vi "Generate.vi"(8 "error in (no error)":errorcluster, 10 "PCL Rate (secs)":dbl, 11 "Frame Configurations":T1[](array[typedef]) {"CD Results Refs"."Data Reference" format="%.0x"; "Input Channels Refs"."Data Reference" format="%.0x"; "Frame Configuration"."CRC"."Data Type" items=["Signed", "Unsigned", "IEEE Float"]; "Frame Configuration"."Rolling Counter"."Data Type" items=["Signed", "Unsigned", "IEEE Float"]; "Frame Configuration"."Input Channels"."Data Type" items=["Signed", "Unsigned", "IEEE Float"]}) -> (0 "error out":errorcluster, 3 "Frame Configurations":T1[](array[typedef]) {"CD Results Refs"."Data Reference" format="%.0x"; "Input Channels Refs"."Data Reference" format="%.0x"; "Frame Configuration"."CRC"."Data Type" items=["Signed", "Unsigned", "IEEE Float"]; "Frame Configuration"."Rolling Counter"."Data Type" items=["Signed", "Unsigned", "IEEE Float"]; "Frame Configuration"."Input Channels"."Data Type" items=["Signed", "Unsigned", "IEEE Float"]})   [LabVIEW 2021, in "LIN Frame Protection Addon Engine.lvlib"]
uses:
  LIN Frame Protection Addon Engine.lvlib
  Types/RT Engine Generate References.ctl
  Shared/Types/FrameConfiguration.ctl
  Shared/Types/InputChannelConfiguration.ctl
  Shared/Types/Protection Type.ctl
  <vilib>/NI VeriStand/Custom Device API/Block Data Reference.ctl
  <vilib>/NI VeriStand/Custom Device API/Data Reference.ctl
  <vilib>/NI VeriStand/Custom Device API/Global Data Refs.vi
  <vilib>/NI VeriStand/Custom Device API/Custom Device API.lvlib
  Shared/LIN Frame Protection Addon Shared.lvlib
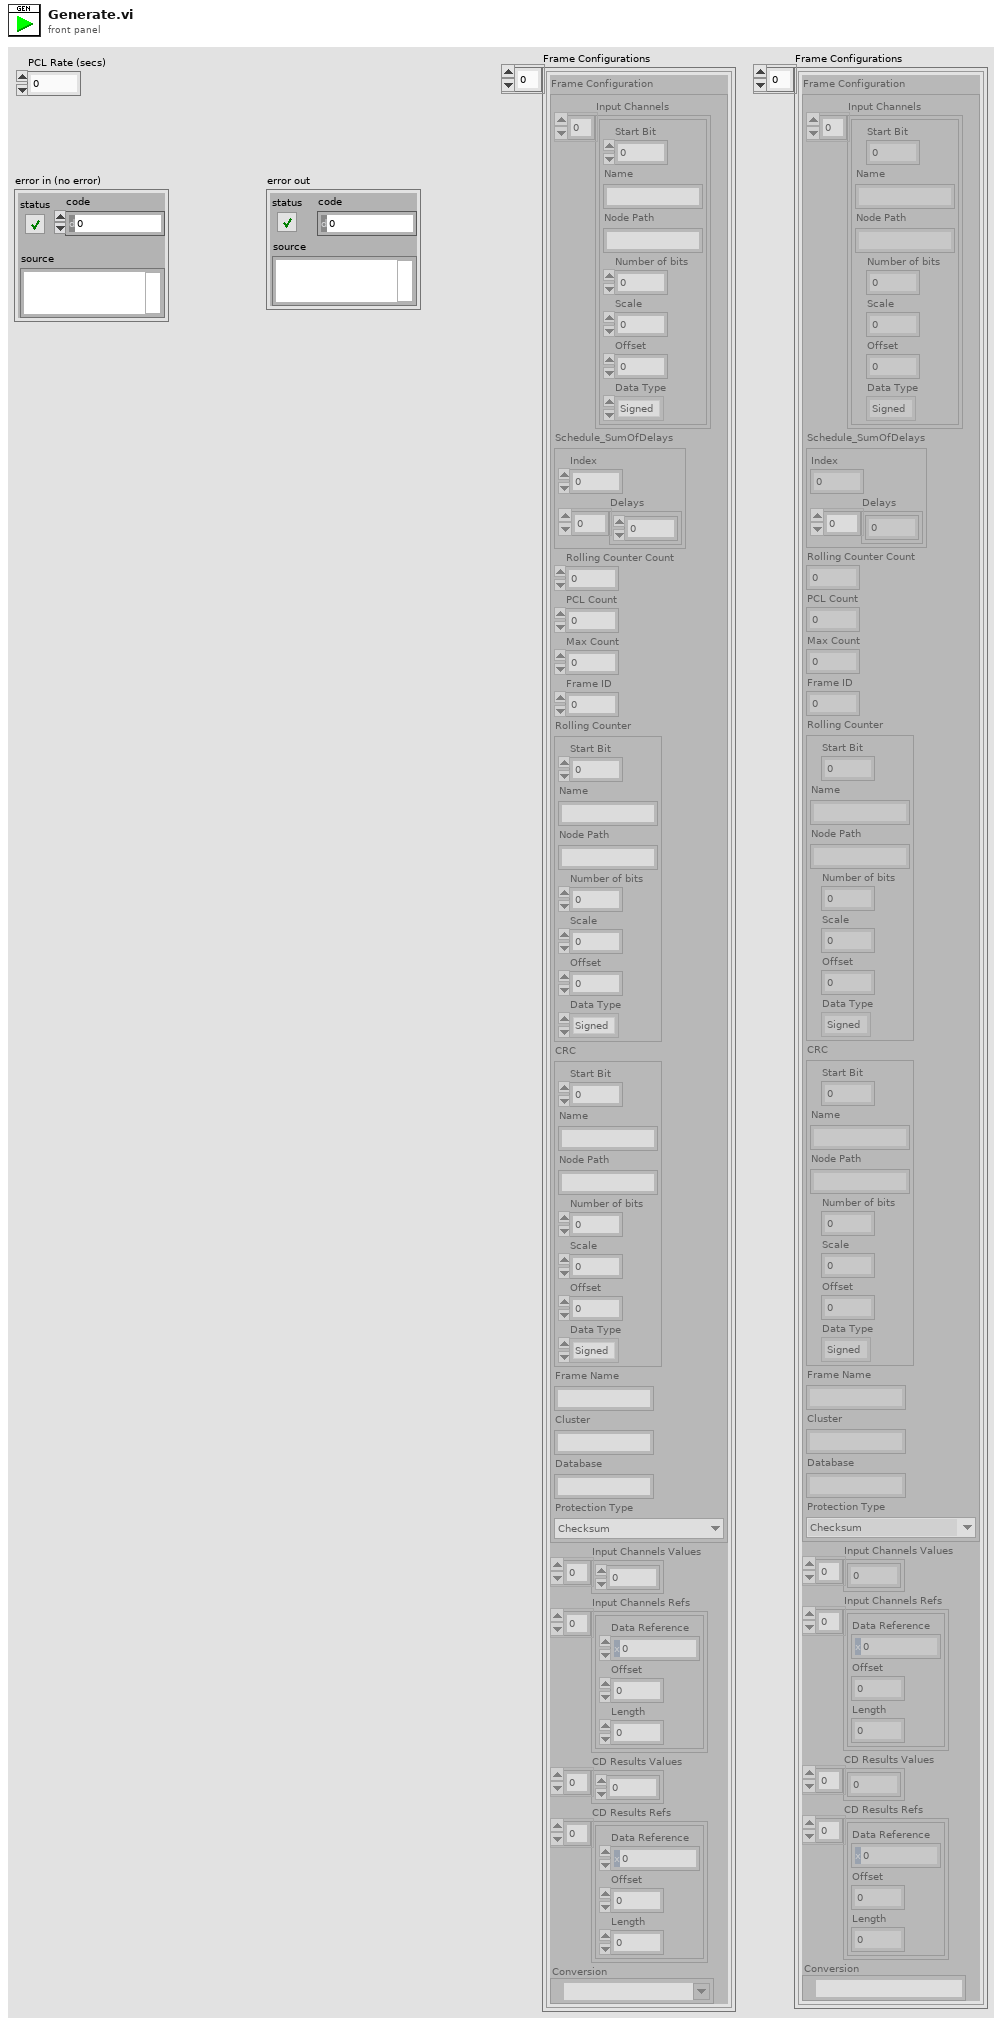
[diagram p1: front panel]
types:
  T1 = typedef "LIN Frame Protection Addon Engine.lvlib/RT Engine Generate References.ctl" = cluster{"Frame Configuration":T2, "Input Channels Values":dbl[], "Input Channels Refs":T5[], "CD Results Values":dbl[], "CD Results Refs":T5[], "Conversion":refnum<k21>}
  T2 = typedef "LIN Frame Protection Addon Shared.lvlib/FrameConfiguration.ctl" = cluster{"Input Channels":T3[], "Schedule_SumOfDelays":cluster{"Index":i32, "Delays":dbl[]}, "Rolling Counter Count":dbl, "PCL Count":u64, "Max Count":dbl, "Frame ID":u32, "Rolling Counter":T3, "CRC":T3, "Frame Name":string, "Cluster":string, "Database":string, "Protection Type":T4}
  T3 = typedef "LIN Frame Protection Addon Shared.lvlib/InputChannelConfiguration.ctl" = cluster{"Start Bit":i32, "Name":string, "Node Path":string, "Number of bits":i32, "Scale":dbl, "Offset":dbl, "Data Type":u32}
  T4 = typedef "LIN Frame Protection Addon Shared.lvlib/Protection Type.ctl" = enum16{"Checksum", "CRC", "None (Counter Only)"}
  T5 = typedef "Custom Device API.lvlib/Block Data Reference.ctl" = cluster{"Data Reference":T6, "Offset":u64, "Length":u64}
  T6 = typedef "Custom Device API.lvlib/Data Reference.ctl" = i32
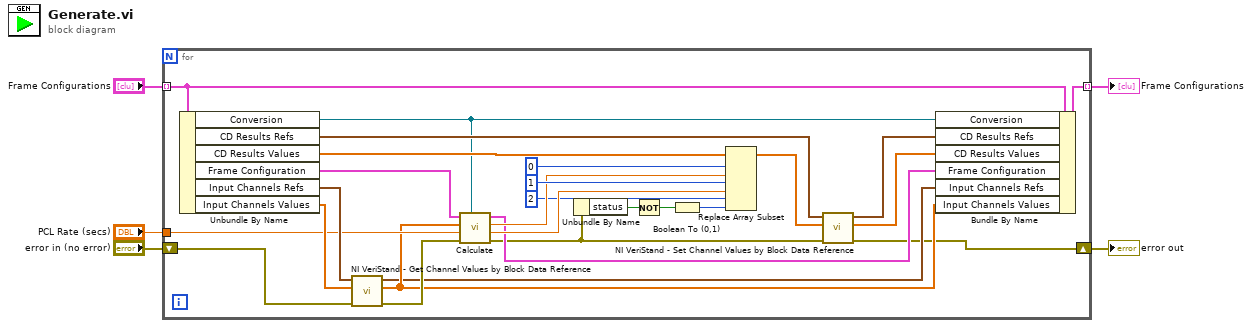
[diagram p0: block diagram]
diagram:
  n1 = for {
    tunnel: "Frame Configurations" -> [w27] mode=indexing
    tunnel: "PCL Rate (secs)" -> [w28]
    shift-right: [w13] -> w2
    shift-left: "error in (no error)" -> [w30]
    tunnel: [w12] -> w4 mode=indexing
    n2 = Unbundle By Name(w27) -> ("Conversion"=w6:refnum<k21>, "CD Results Refs"=w25:T5[], "CD Results Values"=w26:dbl[], "Frame Configuration"=w29:T2, "Input Channels Refs"=w31:T5[], "Input Channels Values"=w32:dbl[])
    n3 = call <vilib>:"NI VeriStand - Get Channel Values by Block Data Reference.vi"("error in (no error)"=w30, "Values Array in"=w32, "Block Data Ref"=w31) -> ("error out"=w19:errorcluster, "Values Array out"=w16:dbl[], "Block Data Ref dup"=w15:T5[])  [unwired: 6 in]
    n4 = call "Calculate.vi"("Conversion"=w6, "error in (no error)"=w19, "PCL dt"=w28, "Values"=w16, "Frame Configuration"=w29) -> ("error out"=w11:errorcluster, "ProtectionValue"=w20:dbl, "Rolling Counter"=w21:dbl, "Frame Configuration"=w14:T2)  [unwired: 3 in]
    n5 = Unbundle By Name(w11) -> ("status"=w10:bool)
    n6 = Not(x=w10) -> (.not. x?=w9:bool)
    n7 = Boolean To (0,1)(Boolean=w9) -> (0, 1=w8:i16)
    n8 = Replace Array Subset(array=w26, new element #1=w21, index #1=0 ("index"), new element #2=w20, index #2=1 ("index"), new element #3=w8, index #3=2 ("index")) -> (w24:dbl[])
    n9 = call <vilib>:"NI VeriStand - Set Channel Values by Block Data Reference.vi"("error in (no error)"=w11, "Values Array in"=w24, "Block Data Ref"=w25) -> ("error out"=w13:errorcluster, "Values Array out"=w17:dbl[], "Block Data Ref dup"=w18:T5[])  [unwired: 6 in]
    n10 = Bundle By Name(cluster=w27, "Conversion"=w6, "CD Results Refs"=w18, "CD Results Values"=w17, "Frame Configuration"=w14, "Input Channels Refs"=w15, "Input Channels Values"=w16) -> (w12:T1)
  }
  "Frame Configurations" <- w4
  "error out" <- w2
